vi "HEWH LaundryNet Tester.vi"() -> ()   [LabVIEW 2016]
uses:
  Utility/LabVIEW GEA2 Toolkit v1.0.0.0/type defs/Data Out.ctl
  Utility/LabVIEW GEA2 Toolkit v1.0.0.0/library/GEA2_Toolkit.lvlib
panel:
  out "Time A":string
  out "Messages A":string[](array[string])
  out "Board ID A":string
  out "Board ID B":string
  out "Board ID C":string
  out "Board ID D":string
  out "Output D, 517":T1 {"CRC" format="%04x"; "Length" format="%02x"; "Command" format="%02x"; "Destination" format="%02x"; "Source" format="%02x"}
  out "Time 4":u32
  out "time stamp 4":timestamp
  out "hex integer string 4":string
  out "Time D":string
  out "Messages D":string[](array[string])
  out "Time Array":u32[](array[numeric])
  out "Error Out 5":errorcluster
  in  "Error In 5":errorcluster
  out "Output C, 521":T1 {"CRC" format="%04x"; "Length" format="%02x"; "Command" format="%02x"; "Destination" format="%02x"; "Source" format="%02x"}
  out "Time 3":u32
  out "time stamp 3":timestamp
  out "hex integer string 3":string
  out "Time C":string
  out "Messages C":string[](array[string])
  out "Error Out 4":errorcluster
  in  "Error In 4":errorcluster
  out "Output 51D, B":T1 {"CRC" format="%04x"; "Length" format="%02x"; "Command" format="%02x"; "Destination" format="%02x"; "Source" format="%02x"}
  out "Time 2":u32
  out "time stamp 2":timestamp
  out "hex integer string 2":string
  out "Time B":string
  out "Messages B":string[](array[string])
  out "Error Out 3":errorcluster
  in  "Error In 3":errorcluster
  out "Output 535, A":T1 {"CRC" format="%04x"; "Length" format="%02x"; "Command" format="%02x"; "Destination" format="%02x"; "Source" format="%02x"}
  out "Time":u32
  out "time stamp":timestamp
  out "hex integer string":string
  out "Error Out 2":errorcluster
  in  "Error In 2":errorcluster
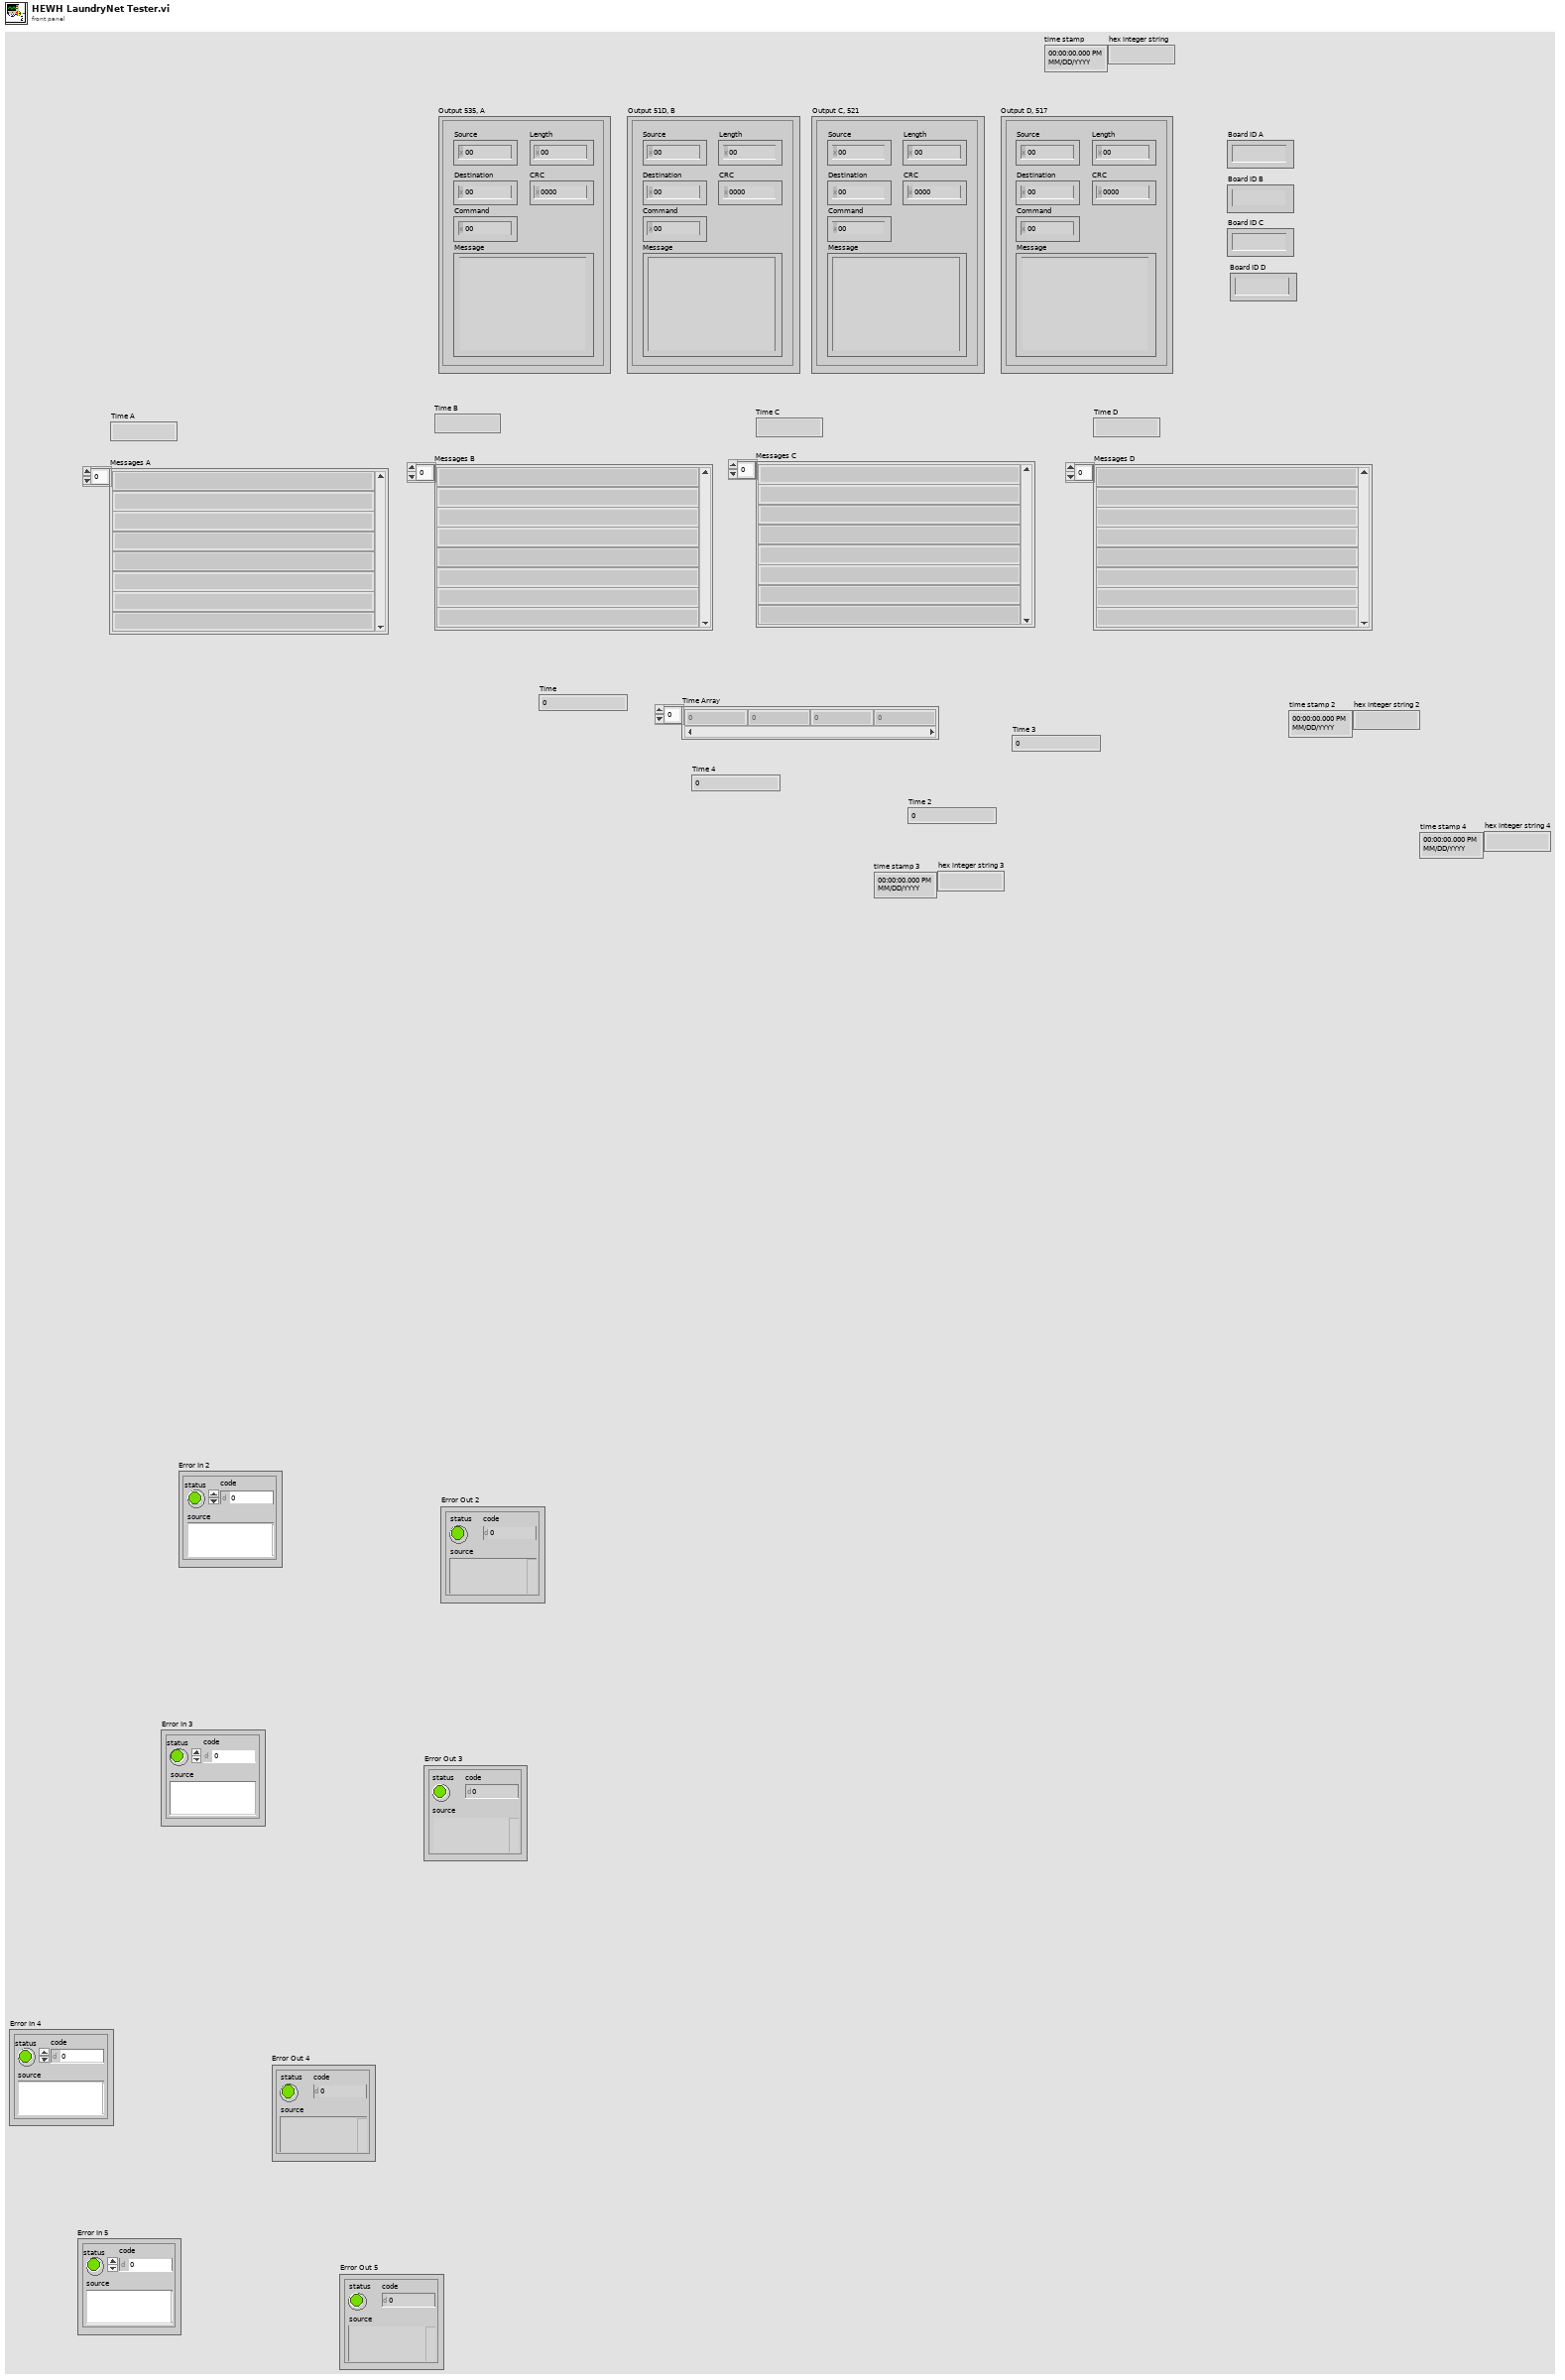
[diagram p1: front panel]
types:
  T1 = typedef "GEA2_Toolkit.lvlib/Data Out.ctl" = cluster{"Source":u8, "Destination":u8, "Command":u8, "Length":u8, "CRC":u16, "Message":string}
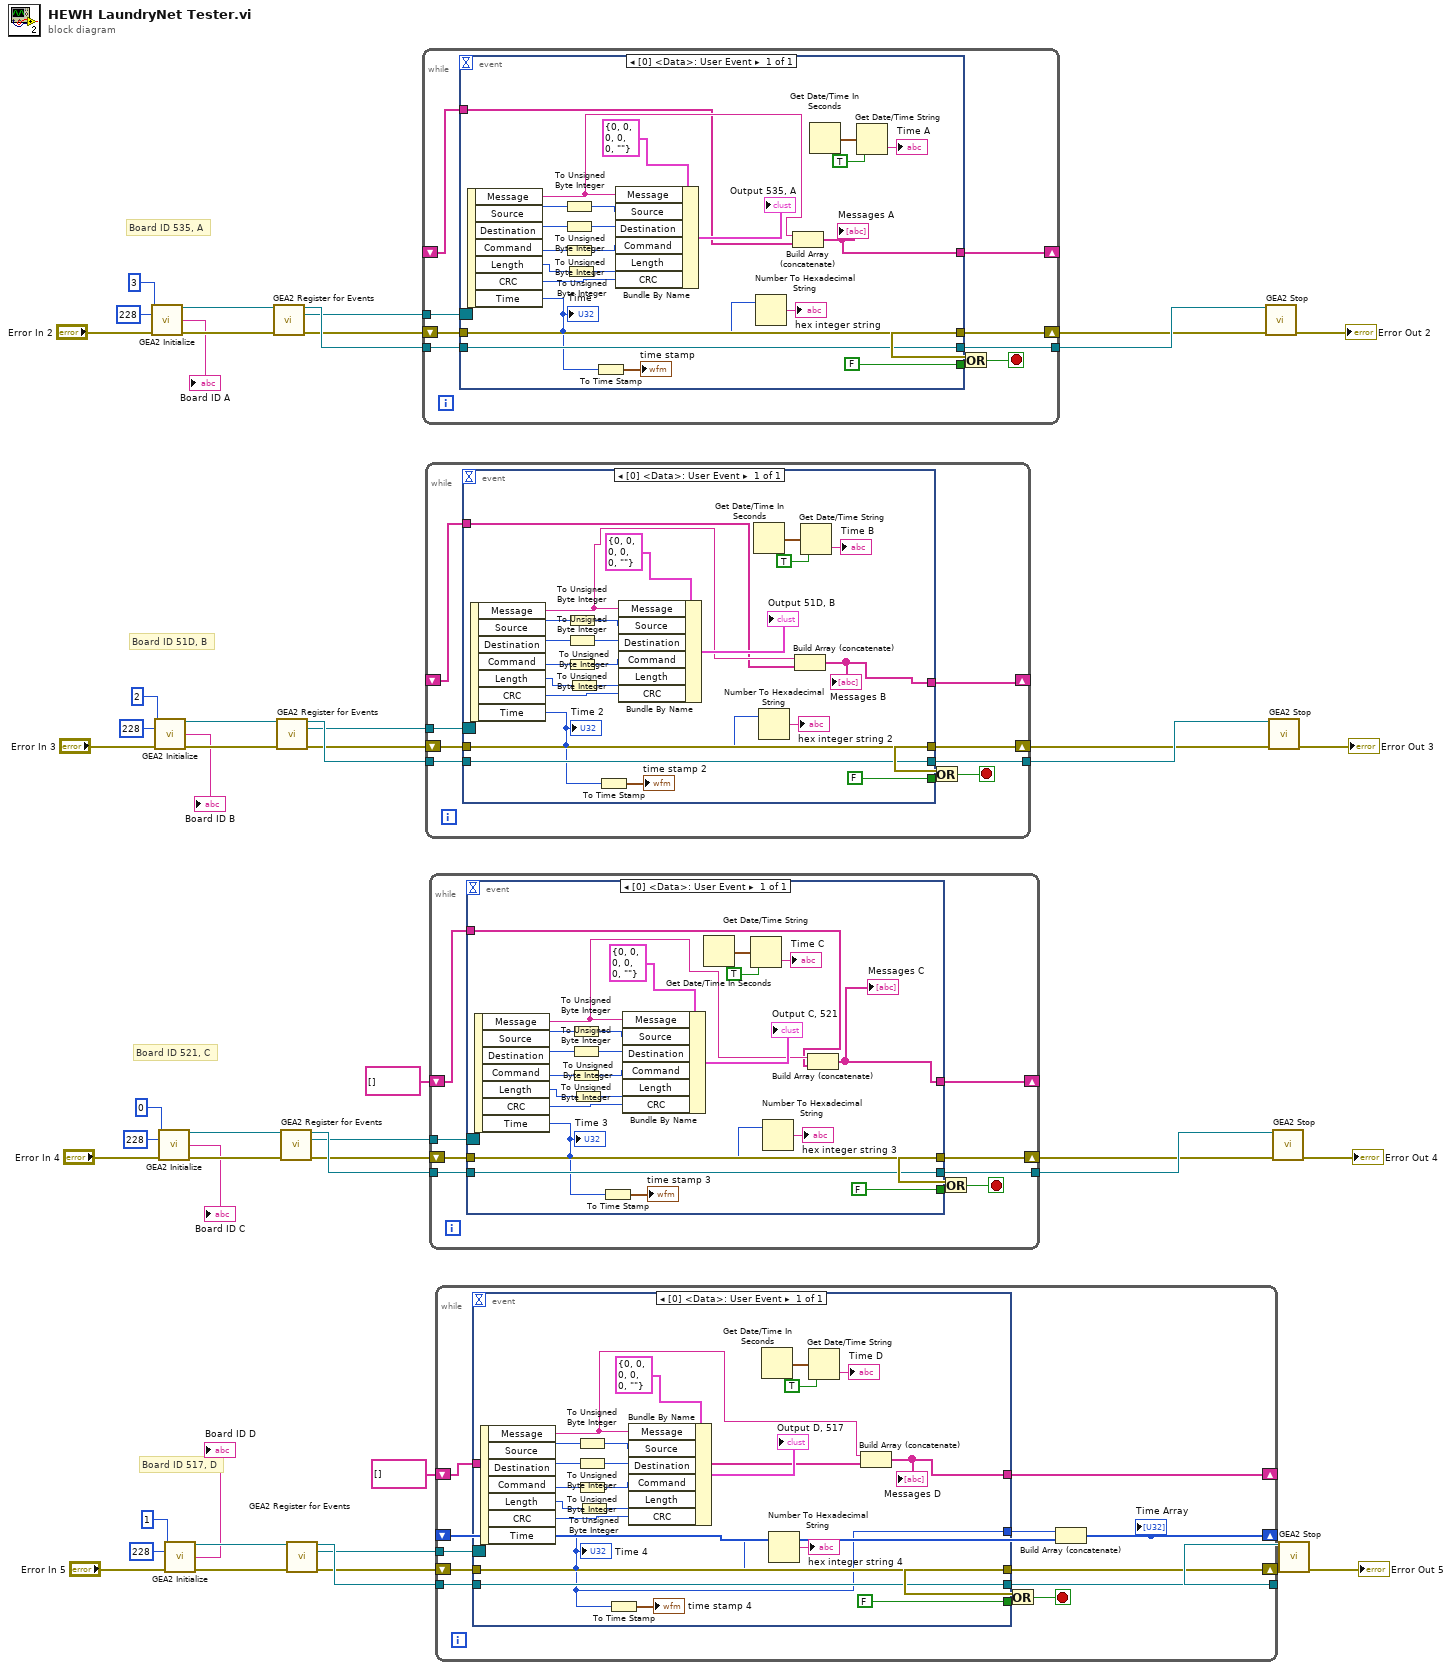
[diagram p0: block diagram]
diagram:
  # "Board ID 517, D"
  # "Board ID 521, C"
  # "Board ID 51D, B"
  # "Board ID 535, A"
  n1 = call "GEA2 Initialize.vi"("Board Index"=3, "Source Address"=u8 228, "error in"="Error In 2") -> ("GEA2 Reference Out"=w48:refnum<k24>, "Board ID"=→"Board ID A":string, "error out"=w49:errorcluster)  [unwired: 10 in]
  n2 = call "GEA2 Initialize.vi"("Board Index"=2, "Source Address"=u8 228, "error in"="Error In 3") -> ("GEA2 Reference Out"=w37:refnum<k24>, "Board ID"=→"Board ID B":string, "error out"=w38:errorcluster)  [unwired: 10 in]
  n3 = call "GEA2 Initialize.vi"("Board Index"=0, "Source Address"=u8 228, "error in"="Error In 4") -> ("GEA2 Reference Out"=w26:refnum<k24>, "Board ID"=→"Board ID C":string, "error out"=w27:errorcluster)  [unwired: 10 in]
  n4 = call "GEA2 Initialize.vi"("Board Index"=1, "Source Address"=u8 228, "error in"="Error In 5") -> ("GEA2 Reference Out"=w15:refnum<k24>, "Board ID"=→"Board ID D":string, "error out"=w16:errorcluster)  [unwired: 10 in]
  n5 = call "GEA2 Register for Events.vi"("GEA2 Reference In"=w48, "Error In"=w49) -> ("GEA2 Reference Out"=w44:refnum<k24>, "GEA2 Event Registration"=w42:refnum<event-registration>, "Error Out"=w43:errorcluster)  [unwired: 11 in]
  n6 = call "GEA2 Register for Events.vi"("GEA2 Reference In"=w37, "Error In"=w38) -> ("GEA2 Reference Out"=w33:refnum<k24>, "GEA2 Event Registration"=w31:refnum<event-registration>, "Error Out"=w32:errorcluster)  [unwired: 11 in]
  n7 = call "GEA2 Register for Events.vi"("GEA2 Reference In"=w26, "Error In"=w27) -> ("GEA2 Reference Out"=w22:refnum<k24>, "GEA2 Event Registration"=w20:refnum<event-registration>, "Error Out"=w21:errorcluster)  [unwired: 11 in]
  n8 = call "GEA2 Register for Events.vi"("GEA2 Reference In"=w15, "Error In"=w16) -> ("GEA2 Reference Out"=w11:refnum<k24>, "GEA2 Event Registration"=w9:refnum<event-registration>, "Error Out"=w10:errorcluster)  [unwired: 11 in]
  n9 = while {
    tunnel: w42 -> [w58]
    tunnel: [w55] -> w47
    tunnel: w44 -> [w56]
    shift-right: [w54] -> w46
    shift-left: w43 -> [w57]
    shift-right: [w52] -> _
    shift-left: _ -> [w51]
    stop <- w59 stop-if-true
    n10 = event shown="[0] <Data>: User Event" {
      selector: w58 -> [_]
      dyn-events: _ -> [_]
      timeout: _ -> [_]
      tunnel: w57 -> [w70]
      tunnel: [w70] -> w54
      tunnel: w56 -> [w79]
      tunnel: [w79] -> w55
      tunnel: [FALSE ("Stop")] -> w53
      tunnel: [w64] -> w52
      tunnel: w51 -> [w63]
      event User Event {
        n11 = event-data() -> ("Message"=w65:string, "Source"=w80:u8, "Destination"=w81:u8, "Command"=w82:u8, "Length"=w75:u8, "CRC"=w69:u16, "Time"=w67:u32)  [unwired: 1 in]
        "Time" <- w67
        n12 = To Unsigned Byte Integer(number=w80) -> (unsigned 8bit integer=w74:u8)
        n13 = To Unsigned Byte Integer(number=w81) -> (unsigned 8bit integer=w73:u8)
        n14 = To Unsigned Byte Integer(number=w82) -> (unsigned 8bit integer=w72:u8)
        n15 = To Unsigned Byte Integer(number=w75) -> (unsigned 8bit integer=w76:u8)
        n16 = To Time Stamp(1:w67) -> (0:→"time stamp":timestamp)
        n17 = Bundle By Name(cluster=T1 {"Source"=0, "Destination"=0, "Command"=0, "Length"=0, "CRC"=0, "Message"=""} ("Data Out"), "Message"=w65, "Source"=w74, "Destination"=w73, "Command"=w72, "Length"=w76, "CRC"=w69) -> (→"Output 535, A":T1)
        n18 = Number To Hexadecimal String(2:w67) -> (0:→"hex integer string":string)  [unwired: 1 in]
        n19 = Build Array (concatenate)(w65, w63) -> (w64:string[])
        "Messages A" <- w64
        n20 = Get Date/Time In Seconds() -> (seconds since 1Jan1904=w62:timestamp)
        n21 = Get Date/Time String(seconds (now)=w62, want seconds? (F)=TRUE) -> (time string=→"Time A":string)  [unwired: 1 in, 1 out]
      }
    }
    n22 = Or(x=w54, y=w53) -> (x .or. y?=w59:bool)
  }
  n23 = while {
    tunnel: w31 -> [w90]
    tunnel: [w87] -> w36
    tunnel: w33 -> [w88]
    shift-right: [w86] -> w35
    shift-left: w32 -> [w89]
    shift-right: [w84] -> _
    shift-left: _ -> [w83]
    stop <- w91 stop-if-true
    n24 = event shown="[0] <Data>: User Event" {
      selector: w90 -> [_]
      dyn-events: _ -> [_]
      timeout: _ -> [_]
      tunnel: w89 -> [w102]
      tunnel: [w102] -> w86
      tunnel: w88 -> [w111]
      tunnel: [w111] -> w87
      tunnel: [FALSE ("Stop")] -> w85
      tunnel: [w93] -> w84
      tunnel: w83 -> [w92]
      event User Event {
        n25 = event-data() -> ("Message"=w94:string, "Source"=w112:u8, "Destination"=w113:u8, "Command"=w114:u8, "Length"=w107:u8, "CRC"=w101:u16, "Time"=w99:u32)  [unwired: 1 in]
        "Time 2" <- w99
        n26 = To Unsigned Byte Integer(number=w112) -> (unsigned 8bit integer=w106:u8)
        n27 = To Unsigned Byte Integer(number=w113) -> (unsigned 8bit integer=w105:u8)
        n28 = To Unsigned Byte Integer(number=w114) -> (unsigned 8bit integer=w104:u8)
        n29 = To Unsigned Byte Integer(number=w107) -> (unsigned 8bit integer=w108:u8)
        n30 = To Time Stamp(1:w99) -> (0:→"time stamp 2":timestamp)
        n31 = Bundle By Name(cluster=T1 {"Source"=0, "Destination"=0, "Command"=0, "Length"=0, "CRC"=0, "Message"=""} ("Data Out"), "Message"=w94, "Source"=w106, "Destination"=w105, "Command"=w104, "Length"=w108, "CRC"=w101) -> (→"Output 51D, B":T1)
        n32 = Get Date/Time In Seconds() -> (seconds since 1Jan1904=w97:timestamp)
        n33 = Number To Hexadecimal String(2:w99) -> (0:→"hex integer string 2":string)  [unwired: 1 in]
        n34 = Build Array (concatenate)(w94, w92) -> (w93:string[])
        "Messages B" <- w93
        n35 = Get Date/Time String(seconds (now)=w97, want seconds? (F)=TRUE) -> (time string=→"Time B":string)  [unwired: 1 in, 1 out]
      }
    }
    n36 = Or(x=w86, y=w85) -> (x .or. y?=w91:bool)
  }
  n37 = while {
    tunnel: w20 -> [w122]
    tunnel: [w119] -> w25
    tunnel: w22 -> [w120]
    shift-right: [w118] -> w24
    shift-left: w21 -> [w121]
    shift-right: [w116] -> _
    shift-left: string[] [] -> [w115]
    stop <- w123 stop-if-true
    n38 = event shown="[0] <Data>: User Event" {
      selector: w122 -> [_]
      dyn-events: _ -> [_]
      timeout: _ -> [_]
      tunnel: w121 -> [w134]
      tunnel: [w134] -> w118
      tunnel: w120 -> [w143]
      tunnel: [w143] -> w119
      tunnel: [FALSE ("Stop")] -> w117
      tunnel: [w125] -> w116
      tunnel: w115 -> [w124]
      event User Event {
        n39 = event-data() -> ("Message"=w126:string, "Source"=w144:u8, "Destination"=w145:u8, "Command"=w146:u8, "Length"=w139:u8, "CRC"=w133:u16, "Time"=w131:u32)  [unwired: 1 in]
        "Time 3" <- w131
        n40 = To Unsigned Byte Integer(number=w144) -> (unsigned 8bit integer=w138:u8)
        n41 = To Unsigned Byte Integer(number=w145) -> (unsigned 8bit integer=w137:u8)
        n42 = To Unsigned Byte Integer(number=w146) -> (unsigned 8bit integer=w136:u8)
        n43 = To Unsigned Byte Integer(number=w139) -> (unsigned 8bit integer=w140:u8)
        n44 = To Time Stamp(1:w131) -> (0:→"time stamp 3":timestamp)
        n45 = Bundle By Name(cluster=T1 {"Source"=0, "Destination"=0, "Command"=0, "Length"=0, "CRC"=0, "Message"=""} ("Data Out"), "Message"=w126, "Source"=w138, "Destination"=w137, "Command"=w136, "Length"=w140, "CRC"=w133) -> (→"Output C, 521":T1)
        n46 = Get Date/Time In Seconds() -> (seconds since 1Jan1904=w129:timestamp)
        n47 = Get Date/Time String(seconds (now)=w129, want seconds? (F)=TRUE) -> (time string=→"Time C":string)  [unwired: 1 in, 1 out]
        n48 = Number To Hexadecimal String(2:w131) -> (0:→"hex integer string 3":string)  [unwired: 1 in]
        n49 = Build Array (concatenate)(w126, w124) -> (w125:string[])
        "Messages C" <- w125
      }
    }
    n50 = Or(x=w118, y=w117) -> (x .or. y?=w123:bool)
  }
  n51 = while {
    tunnel: w9 -> [w157]
    tunnel: [w154] -> w14
    tunnel: w11 -> [w155]
    shift-right: [w153] -> w13
    shift-left: w10 -> [w156]
    shift-right: [w148] -> _
    shift-left: string[] [] -> [w147]
    shift-right: [w150] -> _
    shift-left: _ -> [w149]
    stop <- w158 stop-if-true
    n52 = event shown="[0] <Data>: User Event" {
      selector: w157 -> [_]
      dyn-events: _ -> [_]
      timeout: _ -> [_]
      tunnel: w156 -> [w170]
      tunnel: [w170] -> w153
      tunnel: w155 -> [w178]
      tunnel: [w178] -> w154
      tunnel: [FALSE ("Stop")] -> w152
      tunnel: [w159] -> w148
      tunnel: [w165] -> w151
      tunnel: w147 -> [w160]
      event User Event {
        n53 = event-data() -> ("Message"=w161:string, "Source"=w179:u8, "Destination"=w180:u8, "Command"=w181:u8, "Length"=w174:u8, "CRC"=w169:u16, "Time"=w165:u32)  [unwired: 1 in]
        "Time 4" <- w165
        n54 = To Unsigned Byte Integer(number=w179) -> (unsigned 8bit integer=w173:u8)
        n55 = To Unsigned Byte Integer(number=w180) -> (unsigned 8bit integer=w172:u8)
        n56 = To Unsigned Byte Integer(number=w181) -> (unsigned 8bit integer=w171:u8)
        n57 = To Unsigned Byte Integer(number=w174) -> (unsigned 8bit integer=w175:u8)
        n58 = To Time Stamp(1:w165) -> (0:→"time stamp 4":timestamp)
        n59 = Bundle By Name(cluster=T1 {"Source"=0, "Destination"=0, "Command"=0, "Length"=0, "CRC"=0, "Message"=""} ("Data Out"), "Message"=w161, "Source"=w173, "Destination"=w172, "Command"=w171, "Length"=w175, "CRC"=w169) -> (→"Output D, 517":T1)
        n60 = Get Date/Time In Seconds() -> (seconds since 1Jan1904=w164:timestamp)
        n61 = Number To Hexadecimal String(2:w165) -> (0:→"hex integer string 4":string)  [unwired: 1 in]
        n62 = Get Date/Time String(seconds (now)=w164, want seconds? (F)=TRUE) -> (time string=→"Time D":string)  [unwired: 1 in, 1 out]
        n63 = Build Array (concatenate)(w161, w160) -> (w159:string[])
        "Messages D" <- w159
      }
    }
    n64 = Or(x=w153, y=w152) -> (x .or. y?=w158:bool)
    n65 = Build Array (concatenate)(w151, w149) -> (w150:u32[])
    "Time Array" <- w150
  }
  n66 = call "GEA2 Stop.vi"("GEA2 Reference Out"=w47, "Error In"=w46) -> ("Error Out"=→"Error Out 2":errorcluster)  [unwired: 13 in]
  n67 = call "GEA2 Stop.vi"("GEA2 Reference Out"=w36, "Error In"=w35) -> ("Error Out"=→"Error Out 3":errorcluster)  [unwired: 13 in]
  n68 = call "GEA2 Stop.vi"("GEA2 Reference Out"=w25, "Error In"=w24) -> ("Error Out"=→"Error Out 4":errorcluster)  [unwired: 13 in]
  n69 = call "GEA2 Stop.vi"("GEA2 Reference Out"=w14, "Error In"=w13) -> ("Error Out"=→"Error Out 5":errorcluster)  [unwired: 13 in]
